vi "9999.vi"() -> ()   [LabVIEW 2014]
panel:
  in  "Numeric":dbl
  out "output array":dbl[](array[numeric])
  in  "Slide":dbl(slide) scale=0.0..10.0
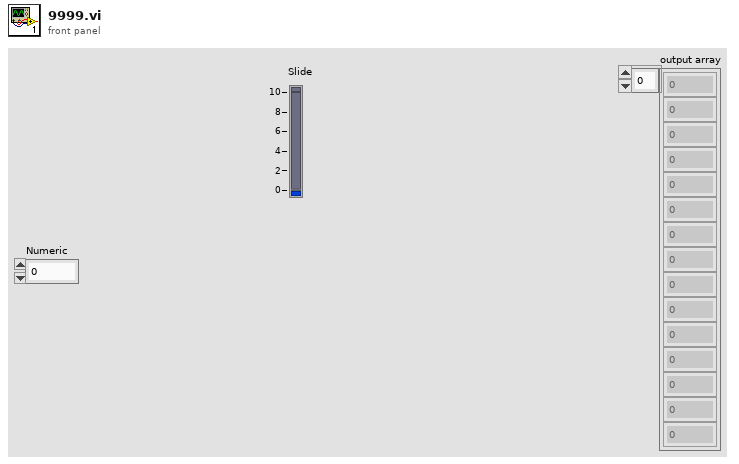
[diagram p1: front panel]
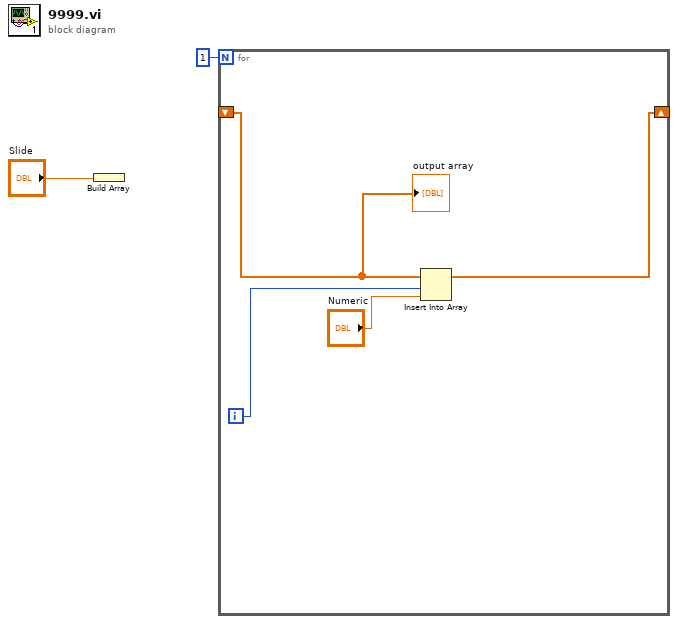
[diagram p0: block diagram]
diagram:
  n1 = Build Array("Slide") -> ()  [unwired: 1 out]
  n2 = for {
    N: 1 -> [_]
    shift-right: [w5] -> _
    shift-left: _ -> [w4]
    i -> [w6]
    n3 = Insert Into Array(array=w4, index=w6, new element="Numeric") -> (w5:dbl[])
    "output array" <- w4
  }
